vi "sub_getNextGuess.vi"(6 "guess candidates":enum16{"level 2 candidates", "all candidates"}(ring), 9 "invalid guesses":T1[](array[typedef]), 10 "current guess queue":T1[](array[typedef]), 11 "solver array":cluster{"solved":bool, "values":string[]}[][](array[cluster])) -> (1 "no valid guess ?":bool, 2 "next guess":T1, 3 "potential guesses":T1[](array[typedef]))   [LabVIEW 2018]
uses:
  guess.ctl
  768c4c62-9cc4-4092-8ce7-16540bf2b464.vi
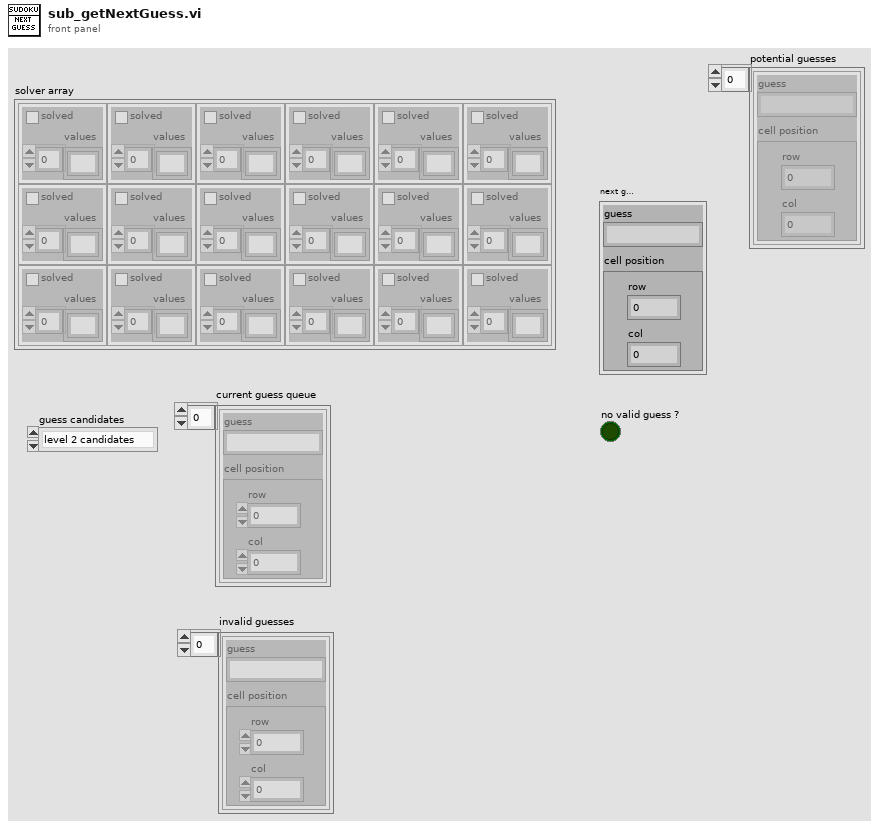
[diagram p1: front panel]
types:
  T1 = typedef "guess.ctl" = cluster{"cell position":cluster{"row":i32, "col":i32}, "guess":string}
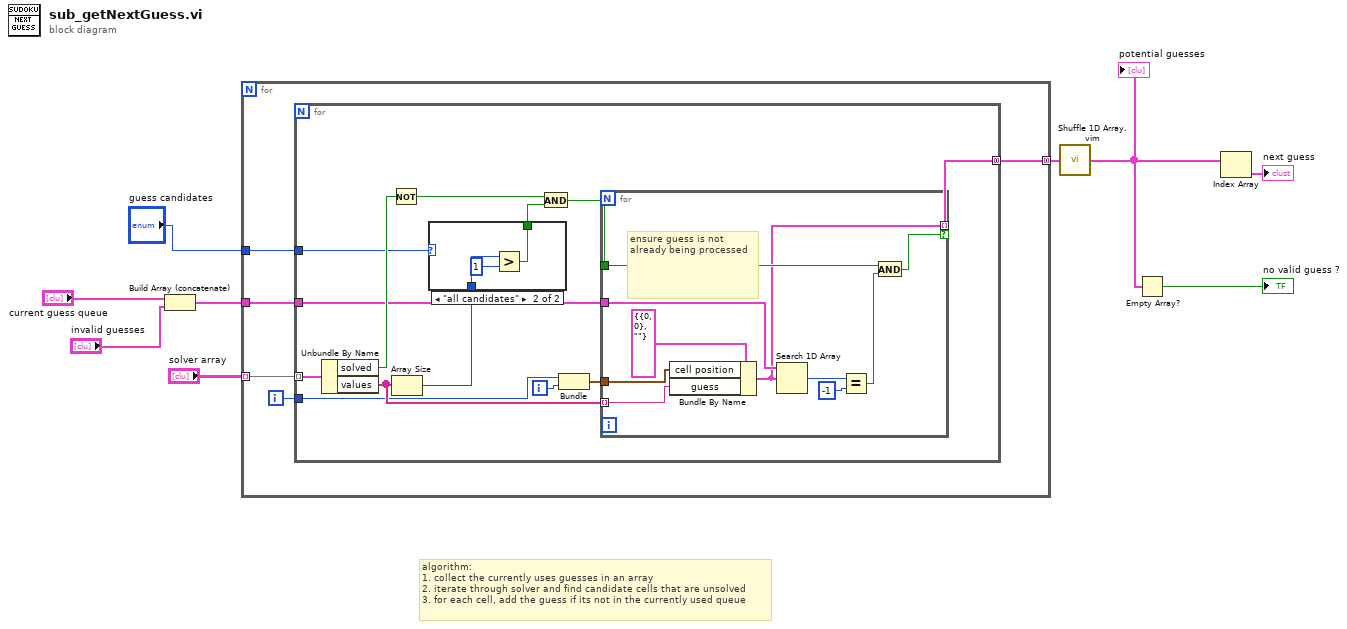
[diagram p0: block diagram]
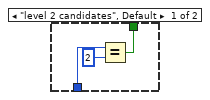
[diagram p2: hidden frame]
diagram:
  # "algorithm:\n1. collect the currently uses guesses in an array\n2. iterate through solver and find candidate cells that are unsolved\n3. for each cell, add the guess if its not in the currently used queue"
  n1 = Build Array (concatenate)("current guess queue", "invalid guesses") -> (w6:T1[])
  n2 = for {
    tunnel: "solver array" -> [w14] mode=indexing
    tunnel: w6 -> [w12]
    tunnel: [w11] -> w3 mode=concatenating
    tunnel: "guess candidates" -> [w10]
    i -> [w13]
    n3 = for {
      tunnel: w14 -> [w27] mode=indexing
      tunnel: w13 -> [w24]
      tunnel: w12 -> [w17]
      tunnel: [w16] -> w11 mode=concatenating
      tunnel: w10 -> [w15]
      i -> [w25]
      n4 = Unbundle By Name(w27) -> ("solved"=w22:bool, "values"=w26:string[])
      n5 = Not(x=w22) -> (.not. x?=w20:bool)
      n6 = Array Size(array=w26) -> (size(s)=w19:i32)
      n7 = case shown="\"all candidates\"" w15 {
        tunnel: w19 -> [w30 w32]
        tunnel: [w28 w33] -> w18
        frame "level 2 candidates", Default {
          n8 = Equal?(x=w30, y=2) -> (x = y?=w28:bool)
        }
        frame "all candidates" {
          n9 = Greater?(x=w32, y=1) -> (0:w33:bool)
        }
      }
      n10 = And(x=w20, y=w18) -> (x .and. y?=w21:bool)
      n11 = Bundle(w24, w25) -> (w23:cluster{i32, i32})  [unwired: 1 in]
      n12 = for {
        tunnel: w26 -> [w41] mode=indexing
        tunnel: w23 -> [w42]
        tunnel: w21 -> [w36]
        tunnel: w17 -> [w40]
        tunnel: [w35] -> w16 mode=indexing if=w34
        # "ensure guess is not \nalready being processed"
        n13 = Bundle By Name(cluster=T1 {"cell position"={"row"=0, "col"=0}, "guess"=""} ("guess"), "cell position"=w42, "guess"=w41) -> (w35:T1)
        n14 = Search 1D Array(1D array=w40, element=w35) -> (index of element=w39:i32)  [unwired: 1 in]
        n15 = Equal?(x=w39, y=-1) -> (x = y?=w37:bool)
        n16 = And(x=w36, y=w37) -> (x .and. y?=w34:bool)
      }
    }
  }
  n17 = call "Shuffle 1D Array.vim"("array"=w3) -> ("shuffled array"=w2:T1[])  [unwired: 4 in]
  "potential guesses" <- w2
  n18 = Empty Array?(array=w2) -> (empty?=→"no valid guess ?":bool)
  n19 = Index Array(array=w2) -> (element=→"next guess":T1)  [unwired: 1 in]
